vi "Decode Base58 UID.vi"(8 "Error In":errorcluster, 11 "Base58 UID":string) -> (0 "Error Out":errorcluster, 3 "UID":u64)   [LabVIEW 2011, in "Tinkerforge.lvlib"]
doc: "This VI decodes the <B>Base58 UID</B> string to the U64 <B>UID</B>."
uses:
  Tinkerforge.lvlib
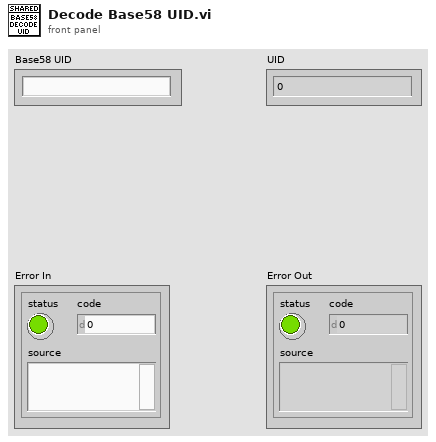
[diagram p1: front panel]
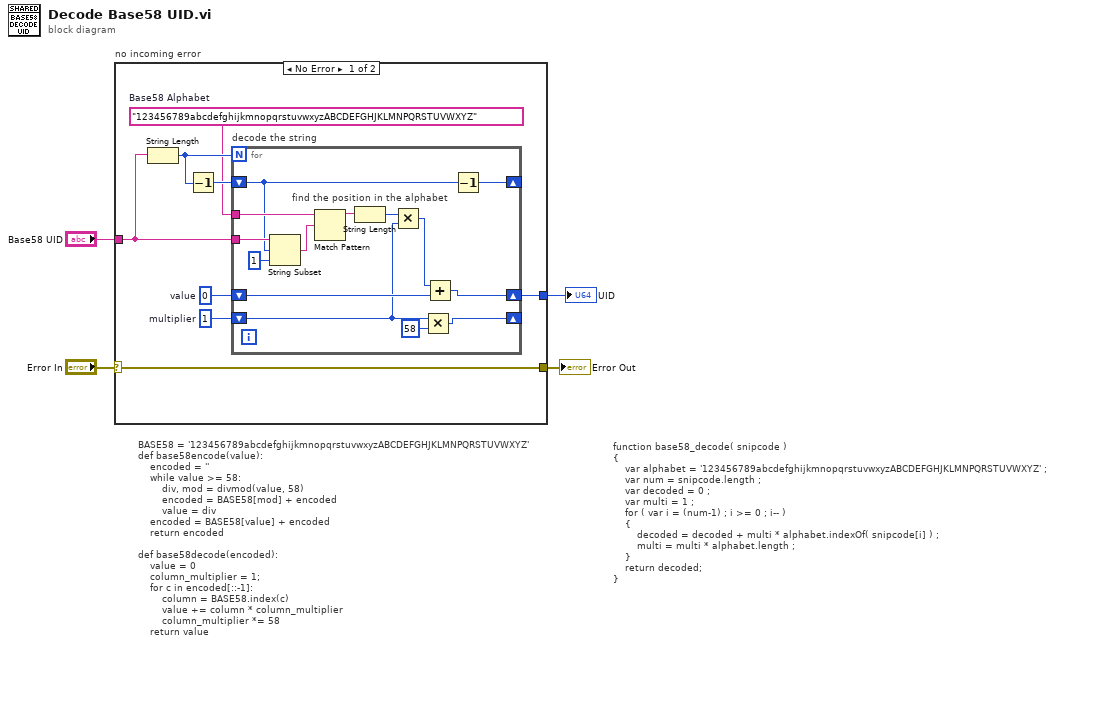
[diagram p0: block diagram]
diagram:
  # "function base58_decode( snipcode )\n{\n    var alphabet = '123456789abcdefghijkmnopqrstuvwxyzABCDEFGHJKLMNPQRSTUVWXYZ' ;\n    var num = snipcode.length ;\n    var decoded = 0 ;\n    var multi = 1 ;\n    for ( var i = (num-1) ; i >= 0 ; i-- )\n    {\n        decoded = decoded + multi * alphabet.indexOf( snipcode[i] ) ;\n        multi = multi * alphabet.length ;\n    }\n    return decoded;\n}"
  # "BASE58 = '123456789abcdefghijkmnopqrstuvwxyzABCDEFGHJKLMNPQRSTUVWXYZ'\ndef base58encode(value):\n    encoded = ''\n    while value >= 58:\n        div, mod = divmod(value, 58)\n        encoded = BASE58[mod] + encoded \n        value = div\n    encoded = BASE58[value] + encoded \n    return encoded\n\ndef base58decode(encoded):\n    value = 0\n    column_multiplier = 1;\n    for c in encoded[::-1]:\n        column = BASE58.index(c)\n        value += column * column_multiplier\n        column_multiplier *= 58\n    return value"
  n1 = case "no incoming error" shown="No Error" "Error In" {
    selector: "Error In" -> [w12 w27]
    tunnel: [w12 w27] -> w3
    tunnel: "Base58 UID" -> [w11 _]
    tunnel: [w5 _] -> w1
    frame No Error {
      w6 = "123456789abcdefghijkmnopqrstuvwxyzABCDEFGHJKLMNPQRSTUVWXYZ"  # Base58 Alphabet
      w7 = u64 1  # multiplier
      w8 = u64 0  # value
      n2 = String Length(string=w11) -> (length=w10:i32)
      n3 = Decrement(x=w10) -> (x-1=w9:i32)
      n4 = for "decode the string" {
        N: w10 -> [_]
        tunnel: w11 -> [w24]
        shift-right: [w26] -> _
        shift-left: w9 -> [w23]
        shift-right: [w16] -> w5
        shift-left: w8 -> [w17]
        shift-right: [w14] -> _
        shift-left: w7 -> [w15]
        tunnel: w6 -> [w25]
        # "find the position in the alphabet"
        n5 = String Subset(string=w24, offset (0)=w23, length (rest)=1 ("length (rest)")) -> (substring=w21:string)
        n6 = Match Pattern(string=w25, regular expression=w21) -> (before substring=w20:string)  [unwired: 1 in, 3 out]
        n7 = String Length(string=w20) -> (length=w19:i32)
        n8 = Multiply(x=w19, y=w15) -> (x*y=w18:u64)
        n9 = Multiply(x=w15, y=u64 58) -> (x*y=w14:u64)
        n10 = Add(x=w18, y=w17) -> (x+y=w16:u64)
        n11 = Decrement(x=w23) -> (x-1=w26:i32)
      }
    }
    frame Error {
    }
  }
  "Error Out" <- w3
  "UID" <- w1
